vi "Logger Open.vi"(8 "error in (no error)":errorcluster, 10 "Queue Name":string) -> (0 "Logger Error Out":errorcluster, 2 "Queue Name Out":string, 3 "LoggerRef Out":T1)   [LabVIEW 2014]
uses:
  LoggerRef.ctl
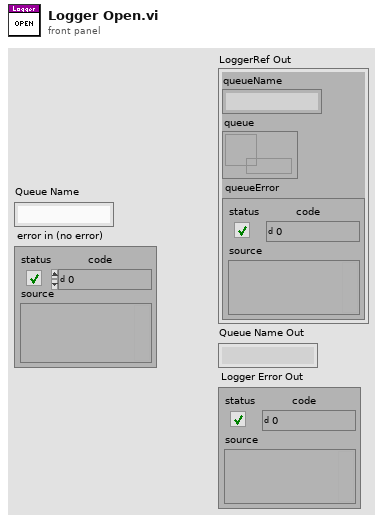
[diagram p1: front panel]
types:
  T1 = typedef "LoggerRef.ctl" = cluster{"queueName":string, "queue":refnum<queue>, "queueError":errorcluster}
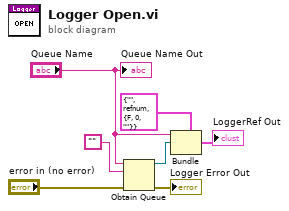
[diagram p0: block diagram]
diagram:
  n1 = Obtain Queue(name (unnamed)="Queue Name", element data type="", error in (no error)="error in (no error)") -> (queue out=w3:refnum<queue>, error out=→"Logger Error Out":errorcluster)  [unwired: 2 in, 1 out]
  n2 = Bundle(cluster=T1 {"queueName"="", "queue"=refnum, "queueError"={"status"=FALSE, "code"=0, "source"=""}} ("LoggerDevRef"), "queueName"="Queue Name", "queue"=w3) -> (→"LoggerRef Out":T1)  [unwired: 1 in]
  "Queue Name Out" <- "Queue Name"
